vi "Laser Feedback_notyet.vi"() -> ()   [LabVIEW 2014]
uses:
  <vilib>/Analysis/polynomials.llb/Scalar Polynomial Evaluation (DBL).vi
  <vilib>/addons/control/pid/pid.llb/PID (DBL).vi
  <vilib>/Analysis/NI_AALPro.lvlib
  <vilib>/addons/control/pid/NI_PID_pid.lvlib
panel:
  out "latest notification":dbl
  out "Error log 2":string
  in  "Averaging Rate  2":i32=10
  out "x/y":dbl
  in  "milliseconds to wait":u32=1
  in  "output range":cluster{"output high":dbl, "output low":dbl}={"output high"=5.0, "output low"=0.1} {"output low" format="%.2f"; "output high" format="%.2f"}
  out "Waveform Chart":dbl(graph)
  in  "Set Power":dbl=10.0
  in  "PID gains":T1={"proportional gain (Kc)"=-0.005, "integral time (Ti, min)"=0.006999999999999955, "derivative time (Td, min)"=0.0} {"derivative time (Td, min)" format="%.7f"; "integral time (Ti, min)" format="%.7f"; "proportional gain (Kc)" format="%.7f"}
  in  "# of Scan Step":dbl=15.0
  in  "min AOM Volt":dbl=0.1
  in  "Max AOM Volt":dbl=4.6
  out "LaserPower (mW)":dbl
  out "IDN String":string
  out "Sensor SN":string
  out "Sensor Name":string
  out "Sensor Flags":bool[](array[boolean])
  in  "stop":bool
  out "Readout value":dbl format="%^#_9e"
  in  "Timeout [ms]":i32=1000
  in  "Readout Config":string(combo)="POW"
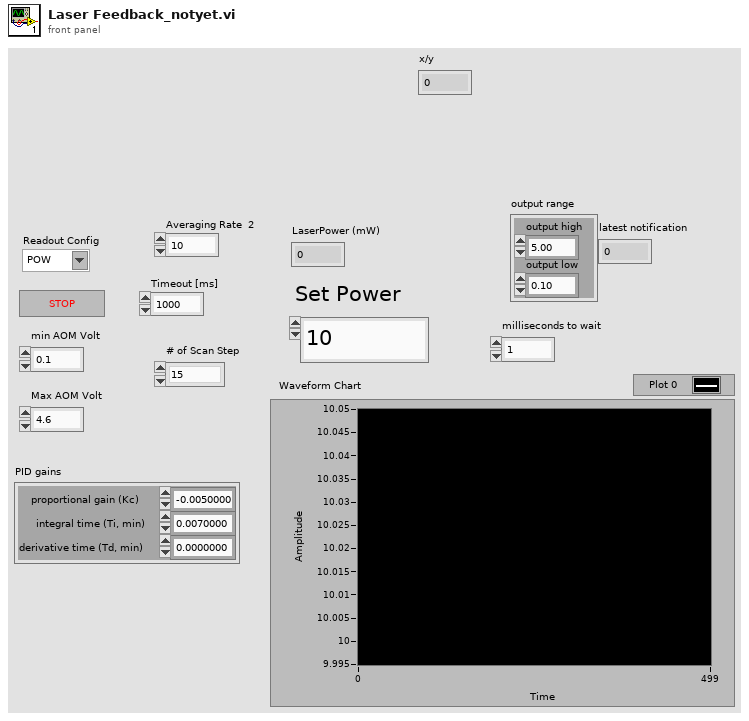
[diagram p1: front panel]
types:
  T1 = cluster{"proportional gain (Kc)":dbl, "integral time (Ti, min)":dbl, "derivative time (Td, min)":dbl}
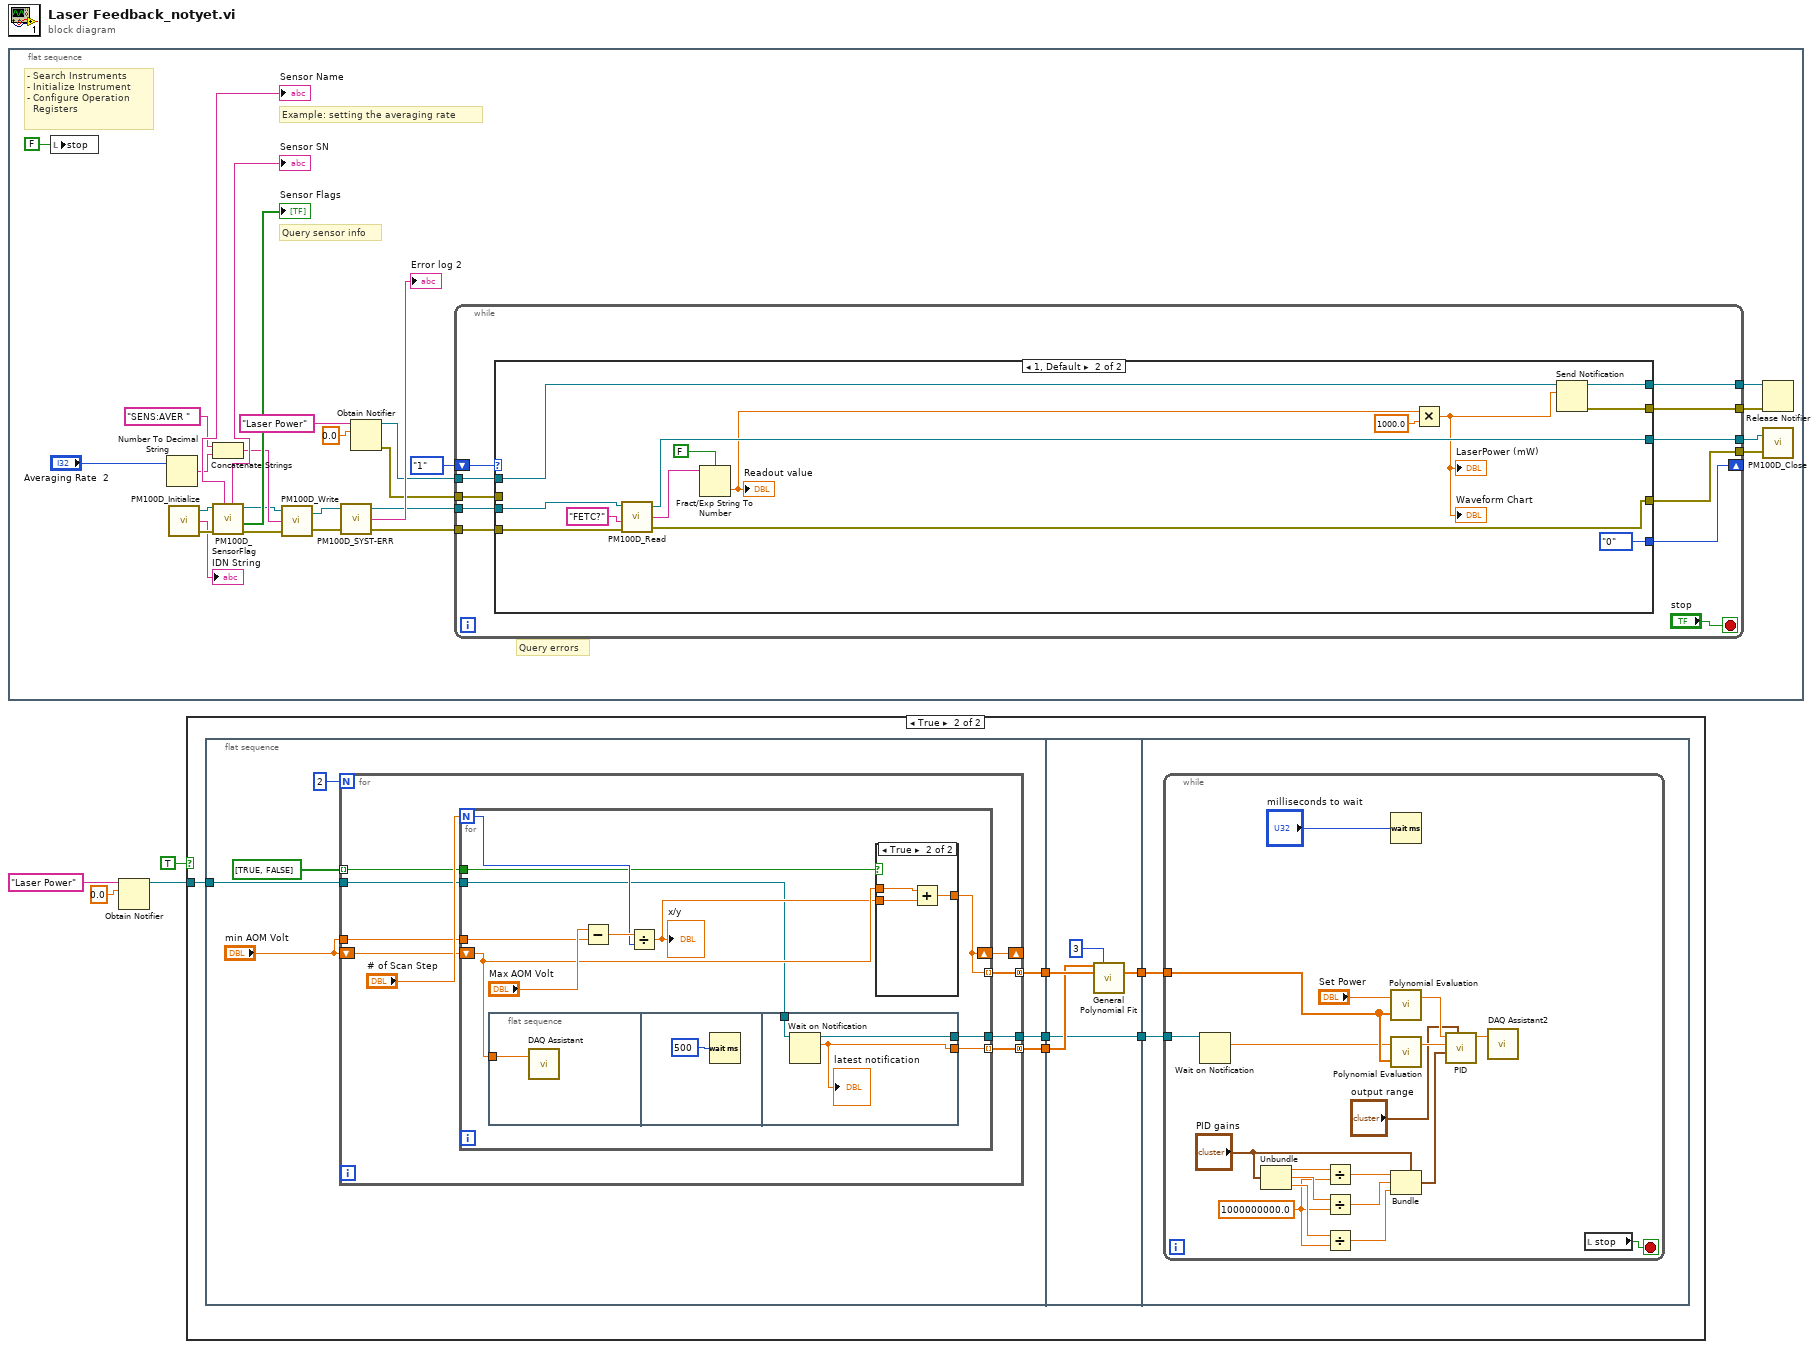
[diagram p0: block diagram]
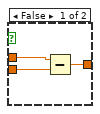
[diagram p3: hidden frame]
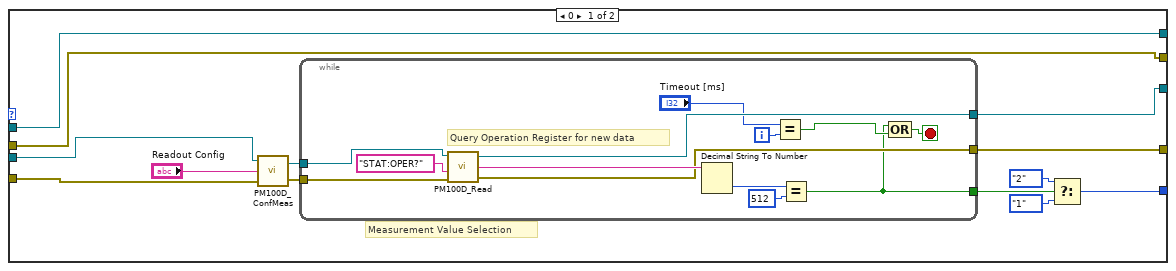
[diagram p4: hidden frame]
diagram:
  n1 = flat-sequence {
    frame #0 {
      # "Query errors"
      # "Example: setting the averaging rate"
      # "- Search Instruments\n- Initialize Instrument\n- Configure Operation\n  Registers"
      # "Query sensor info"
      n2 = local write "stop"(FALSE ("stop")) -> ()
      n3 = Number To Decimal String(number="Averaging Rate  2") -> (decimal integer string=w20:string)  [unwired: 1 in]
      n4 = call "PM100D_Initialize.vi"() -> ("error out"=w30:errorcluster, "Instrument"=→"IDN String":string, "VISA out"=w31:refnum<visa-resource-name>)  [unwired: 2 in, 1 out]
      n5 = Concatenate Strings("SENS:AVER " ("string"), w20) -> (w18:string)
      n6 = call "PM100D_SensorFlag.vi"("error in (no error)"=w30, "VISA in"=w31) -> ("error out"=w13:errorcluster, "flags"=→"Sensor Flags":bool[], "VISA out"=w14:refnum<visa-resource-name>, "sn"=→"Sensor SN":string, "name"=→"Sensor Name":string)  [unwired: 2 in, 3 out]
      n7 = call "PM100D_Write.vi"("error in (no error)"=w13, "Command"=w18, "VISA in"=w14) -> ("error out"=w15:errorcluster, "VISA out"=w17:refnum<visa-resource-name>)
      n8 = call "PM100D_SYST-ERR.vi"("error out 2"=w15, "VISA In"=w17) -> ("error out"=w11:errorcluster, "Error"=→"Error log 2":string, "VISA Out"=w12:refnum<visa-resource-name>)  [unwired: 1 in]
      n9 = Obtain Notifier(name (unnamed)="Laser Power", notification data type=0.0) -> (notifier out=w9:refnum<notifier>, error out=w5:errorcluster)  [unwired: 2 in, 1 out]
      n10 = while {
        tunnel: w12 -> [w42]
        tunnel: w11 -> [w41]
        shift-right: [w38] -> _
        shift-left: enum16{"1", "2"}."1" -> [w39]
        tunnel: [w37] -> w24
        tunnel: [w36] -> w23
        tunnel: w9 -> [w35]
        tunnel: [w34] -> w7
        tunnel: [w33] -> w6
        tunnel: w5 -> [w32]
        stop <- "stop" stop-if-true
        n11 = case shown="1, Default" w39 {
          tunnel: w42 -> [w55 w80]
          tunnel: w41 -> [w54 w79]
          tunnel: [w49 enum16{"0", "1", "2"}."0"] -> w38
          tunnel: [w51 w78] -> w37
          tunnel: [w50 w75] -> w36
          tunnel: w35 -> [w44 w72]
          tunnel: [w44 w70] -> w34
          tunnel: [w43 w69] -> w33
          tunnel: w32 -> [w43 _]
          frame 0 {
            # "Measurement Value Selection"
            n12 = call "PM100D_ConfMeas.vi"("error in"=w54, "Conf:"="Readout Config", "VISA In"=w55) -> ("error out"=w52:errorcluster, "dup VISA session"=w53:refnum<visa-resource-name>)
            n13 = while {
              tunnel: w53 -> [w64]
              tunnel: w52 -> [w63]
              tunnel: [w62] -> w51
              tunnel: [w61] -> w50
              tunnel: [w56] -> w48
              i -> [w58]
              stop <- w60 stop-if-true
              # "Query Operation Register for new data"
              n14 = call "PM100D_Read.vi"("error in (no error)"=w63, "Command"="STAT:OPER?", "VISA in"=w64) -> ("error out"=w61:errorcluster, "ReadValue"=w67:string, "VISA out"=w62:refnum<visa-resource-name>)  [unwired: 1 in]
              n15 = Decimal String To Number(string=w67) -> (number=w66:i32)  [unwired: 2 in, 1 out]
              n16 = Equal?(x="Timeout [ms]", y=w58) -> (x = y?=w57:bool)
              n17 = Equal?(x=w66, y=512) -> (x = y?=w56:bool)
              n18 = Compound Arithmetic op=OR(w56, w57) -> (w60:bool)
            }
            n19 = Select(t=enum16{"1", "2"}."2", s=w48, f=enum16{"1", "2"}."1") -> (s? t:f=w49:enum16{"1", "2"})
          }
          frame 1, Default {
            n20 = call "PM100D_Read.vi"("error in (no error)"=w79, "Command"="FETC?", "VISA in"=w80) -> ("error out"=w75:errorcluster, "ReadValue"=w77:string, "VISA out"=w78:refnum<visa-resource-name>)  [unwired: 1 in]
            n21 = Fract/Exp String To Number(use system decimal point (T)=FALSE, string=w77) -> (number=w74:dbl)  [unwired: 2 in, 1 out]
            "Readout value" <- w74
            n22 = Multiply(x=w74, y=1000.0) -> (x*y=w71:dbl)
            "LaserPower (mW)" <- w71
            "Waveform Chart" <- w71
            n23 = Send Notification(notification=w71, notifier=w72) -> (notifier out=w70:refnum<notifier>, error out=w69:errorcluster)  [unwired: 1 in]
          }
        }
      }
      n24 = Release Notifier(notifier=w7, error in (no error)=w6) -> ()  [unwired: 1 in, 3 out]
      n25 = call "PM100D_Close.vi"("error in (no error)"=w23, "VISA resource name"=w24) -> ()  [unwired: 2 in]
    }
  }
  n26 = Obtain Notifier(name (unnamed)="Laser Power", notification data type=0.0) -> (notifier out=w1:refnum<notifier>)  [unwired: 2 in, 2 out]
  n27 = case shown="True" TRUE {
    tunnel: w1 -> [_ w85]
    frame False {
    }
    frame True {
      n28 = flat-sequence {
        tunnel: [w95] -> w88
        tunnel: [w94] -> w87
        tunnel: w85 -> [w90]
        tunnel: [w89] -> w83
        tunnel: w88 -> [w130]
        tunnel: w87 -> [w129]
        tunnel: [w128] -> w86
        tunnel: [w127] -> w84
        tunnel: w83 -> [w127]
        tunnel: w86 -> [w133]
        tunnel: w84 -> [w132]
        frame #0 {
          n29 = for {
            N: 2 -> [_]
            tunnel: [w103] -> w95 mode=concatenating
            tunnel: [w102] -> w94 mode=concatenating
            shift-right: [w101] -> _
            shift-left: "min AOM Volt" -> [w100]
            tunnel: "min AOM Volt" -> [w99]
            tunnel: bool[] [TRUE, FALSE] -> [w98] mode=indexing
            tunnel: w90 -> [w97]
            tunnel: [w96] -> w89
            n30 = for {
              N: "# of Scan Step" -> [w113]
              tunnel: [w111] -> w103 mode=indexing
              tunnel: [w112] -> w102 mode=indexing
              shift-right: [w111] -> w101
              shift-left: w100 -> [w108]
              tunnel: w99 -> [w110]
              tunnel: w98 -> [w109]
              tunnel: w97 -> [w106]
              tunnel: [w105] -> w96
              n31 = flat-sequence {
                tunnel: w108 -> [w122]
                tunnel: [w125] -> w112
                tunnel: w106 -> [w126]
                tunnel: [w124] -> w105
                frame #0 {
                  n32 = call "DAQ Assistant"("data"=w122) -> ()  [unwired: 17 in, 2 out]
                }
                frame #1 {
                  n33 = Wait (ms)(milliseconds to wait=u32 500) -> ()  [unwired: 1 out]
                }
                frame #2 {
                  n34 = Wait on Notification(notifier=w126) -> (notifier out=w124:refnum<notifier>, notification=w125:dbl)  [unwired: 3 in, 2 out]
                  "latest notification" <- w125
                }
              }
              n35 = Subtract(x="Max AOM Volt", y=w110) -> (x-y=w115:dbl)
              n36 = Divide(x=w115, y=w113) -> (x/y=w107:dbl)
              "x/y" <- w107
              n37 = case shown="True" w109 {
                tunnel: [w116 w121] -> w111
                tunnel: w108 -> [w118 w120]
                tunnel: w107 -> [w117 w119]
                frame False {
                  n38 = Subtract(x=w118, y=w117) -> (x-y=w116:dbl)
                }
                frame True {
                  n39 = Add(x=w120, y=w119) -> (x+y=w121:dbl)
                }
              }
            }
          }
        }
        frame #1 {
          n40 = call <vilib>:"General Polynomial Fit.vi"("Y"=w129, "polynomial order"=3, "X"=w130) -> ("Polynomial Coefficients"=w128:dbl[])  [unwired: 9 in, 3 out]
        }
        frame #2 {
          n41 = while {
            tunnel: w133 -> [w151]
            tunnel: w132 -> [w135]
            stop <- w147 stop-if-true
            w138 = 1000000000.0 ("y")
            n42 = Wait on Notification(notifier=w135) -> (notification=w134:dbl)  [unwired: 3 in, 3 out]
            n43 = Unbundle("PID gains") -> ("proportional gain (Kc)"=w144:dbl, "integral time (Ti, min)"=w143:dbl, "derivative time (Td, min)"=w139:dbl)
            n44 = Divide(x=w144, y=w138) -> (x/y=w141:dbl)
            n45 = Divide(x=w143, y=w138) -> (x/y=w140:dbl)
            n46 = Divide(x=w139, y=w138) -> (x/y=w137:dbl)
            n47 = Wait (ms)(milliseconds to wait="milliseconds to wait") -> ()  [unwired: 1 out]
            n48 = call-poly <vilib>:"Polynomial Evaluation.vi"("P(x)"=w151, "a"="Set Power") -> ("P(a)"=w149:dbl)  [unwired: 1 out]
            n49 = call-poly <vilib>:"Polynomial Evaluation.vi"("P(x)"=w151, "a"=w134) -> ("P(a)"=w150:dbl)  [unwired: 1 out]
            n50 = Bundle(cluster="PID gains", "proportional gain (Kc)"=w141, "integral time (Ti, min)"=w140, "derivative time (Td, min)"=w137) -> (w136:T1)
            n51 = call-poly <vilib>:"PID.vi"("output range"="output range", "PID gains"=w136, "process variable"=w150, "setpoint"=w149) -> ("output"=w148:dbl)  [unwired: 6 in, 1 out]
            n52 = call "DAQ Assistant2"("data"=w148) -> ()  [unwired: 17 in, 2 out]
            n53 = local read "stop"() -> (w147:bool)
          }
        }
      }
    }
  }
